vi "sub_HighPressureWash.vi"(8 "error in":errorcluster caption="에러 입력", 10 "Car Position Slider":refnum<vi>, 11 "Wash Options":refnum<vi>) -> (0 "error out":errorcluster caption="에러 출력", 2 "Elapsed Time (sec)":dbl format="%#.2g", 3 "Wash Indicators":T1)   [LabVIEW 2018]
uses:
  Control/Car Wash Indicators.ctl
  Control/Time.ctl
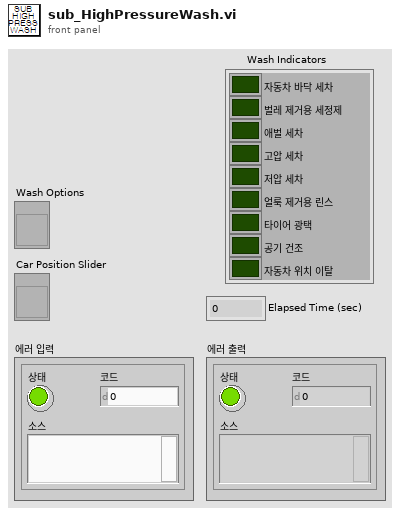
[diagram p1: front panel]
types:
  T1 = typedef "Car Wash Indicators.ctl" = cluster{"자동차 바닥 세차":bool, "벌레 제거용 세정제":bool, "애벌 세차":bool, "고압 세차":bool, "저압 세차":bool, "얼룩 제거용 린스":bool, "타이어 광택":bool, "공기 건조":bool, "자동차 위치 이탈":bool}
  T2 = enum8{"Enabled", "Disabled", "Disabled and Grayed Out"}
  T3 = typedef "Time.ctl" = enum16{"Start", "End"}
  T4 = typedef "Car Position Control.ctl" = i32
  T5 = typedef "Wash Options.ctl" = cluster{"Under Body Wash":bool, "Bug Remover":bool, "Pre-Soak":bool, "High Pressure Wash":bool, "Low Pressure Wax":bool, "Spot Free Rinse":bool, "Tire Shine Foam":bool, "Air Dry":bool}
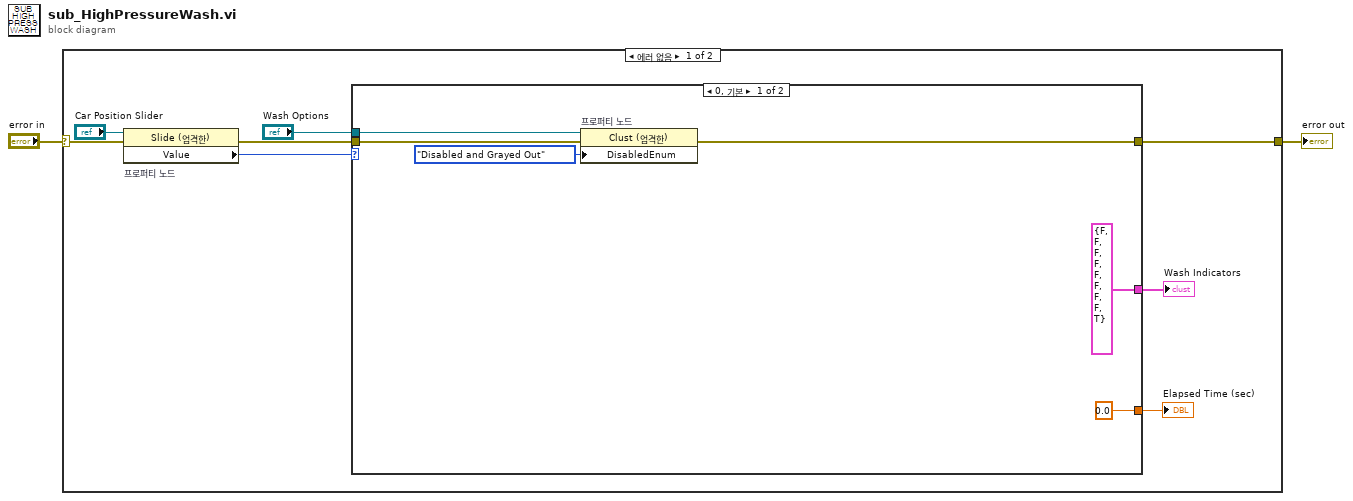
[diagram p0: block diagram]
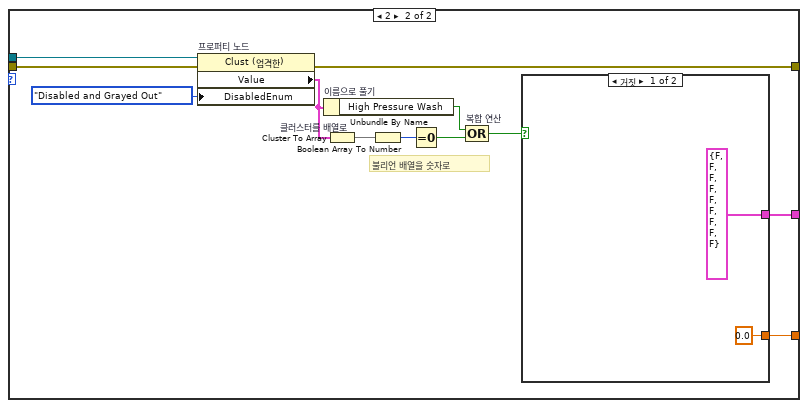
[diagram p2: hidden frame]
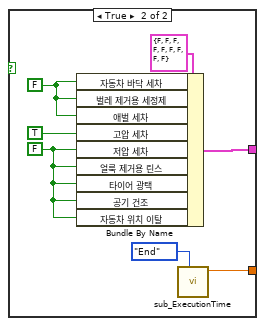
[diagram p3: hidden frame]
diagram:
  n1 = case shown="에러 없음" "error in" {
    selector: "error in" -> [w10 w38]
    tunnel: [w6 w38] -> w1
    frame No Error {
      n2 = property on="프로퍼티 노드" class="Slide (엄격한)"(reference="Car Position Slider", error in=w10) -> (error out=w8:errorcluster, "Value"=w7:T4)  [unwired: 1 out]
      n3 = case shown="0, 기본" w7 {
        tunnel: w8 -> [w14 w28]
        tunnel: [w11 w27] -> w6
        tunnel: [T1 {"자동차 바닥 세차"=FALSE, "벌레 제거용 세정제"=FALSE, "애벌 세차"=FALSE, "고압 세차"=FALSE, "저압 세차"=FALSE, "얼룩 제거용 린스"=FALSE, "타이어 광택"=FALSE, "공기 건조"=FALSE, "자동차 위치 이탈"=TRUE} ("Wash Indicators") w26] -> w5
        tunnel: [0.0 ("Elapsed Time (sec)") w25] -> w4
        tunnel: "Wash Options" -> [w13 w23]
        frame 0, Default {
          n4 = property on="프로퍼티 노드" class="Clust (엄격한)"(reference=w13, error in=w14, "DisabledEnum"=T2."Disabled and Grayed Out" ("비활성화")) -> (error out=w11:errorcluster)  [unwired: 1 out]
        }
        frame 2 {
          # "불리언 배열을 숫자로"
          n5 = property on="프로퍼티 노드" class="Clust (엄격한)"(reference=w23, error in=w28, "DisabledEnum"=T2."Disabled and Grayed Out" ("비활성화")) -> (error out=w27:errorcluster, "Value"=w21:T5)  [unwired: 1 out]
          n6 = Unbundle By Name "이름으로 풀기"(w21) -> ("High Pressure Wash"=w18:bool)
          n7 = Cluster To Array "클러스터를 배열로"(cluster=w21) -> (array=w20:bool[])
          n8 = Boolean Array To Number(Boolean array=w20) -> (number=w22:u32)
          n9 = Equal To 0?(x=w22) -> (x = 0?=w19:bool)
          n10 = Compound Arithmetic op=OR "복합 연산"(w18, w19) -> (w17:bool)
          n11 = case shown="거짓" w17 {
            tunnel: [T1 {"자동차 바닥 세차"=FALSE, "벌레 제거용 세정제"=FALSE, "애벌 세차"=FALSE, "고압 세차"=FALSE, "저압 세차"=FALSE, "얼룩 제거용 린스"=FALSE, "타이어 광택"=FALSE, "공기 건조"=FALSE, "자동차 위치 이탈"=FALSE} ("Wash Indicators") w36] -> w26
            tunnel: [0.0 ("Elapsed Time (sec)") w34] -> w25
            frame False {
            }
            frame True {
              w33 = FALSE ("Under Body Wash")
              w32 = FALSE ("Under Body Wash")
              n12 = Bundle By Name(cluster=T1 {"자동차 바닥 세차"=FALSE, "벌레 제거용 세정제"=FALSE, "애벌 세차"=FALSE, "고압 세차"=FALSE, "저압 세차"=FALSE, "얼룩 제거용 린스"=FALSE, "타이어 광택"=FALSE, "공기 건조"=FALSE, "자동차 위치 이탈"=FALSE} ("Wash Indicators"), "자동차 바닥 세차"=w32, "벌레 제거용 세정제"=w32, "애벌 세차"=w32, "고압 세차"=TRUE ("Under Body Wash"), "저압 세차"=w33, "얼룩 제거용 린스"=w33, "타이어 광택"=w33, "공기 건조"=w33, "자동차 위치 이탈"=w33) -> (w36:T1)
              n13 = call "sub_ExecutionTime.vi"("State"=Time."End") -> ("Elapsed Time (sec)"=w34:dbl)  [unwired: 9 in, 1 out]
            }
          }
        }
      }
      "Wash Indicators" <- w5
      "Elapsed Time (sec)" <- w4
    }
    frame Error {
    }
  }
  "error out" <- w1
